vi "_Find Named Range.vi"(8 "error in":errorcluster, 9 "Sheet Name":string, 10 "Range Identifier":string, 11 "SpreadsheetDocument":refnum<k24>) -> (0 "error out":errorcluster, 1 "End Cell":cluster{"Col":string, "Row":i32}, 2 "Start Cell":cluster{"Col":string, "Row":i32}, 3 "SpreadsheetDocument":refnum<k24>, 4 "Sheet Name":string)   [LabVIEW 2021, in "Open Xml.lvlib"]
uses:
  Open Xml.lvlib
  D:/git/Open-Xml-LabVIEW/DocumentFormat.OpenXml.dll
  DocumentFormat.OpenXml.dll
  D:/git/Open-Xml-LabVIEW/DocumentFormat.OpenXml.Framework.dll
  DocumentFormat.OpenXml.Framework.dll
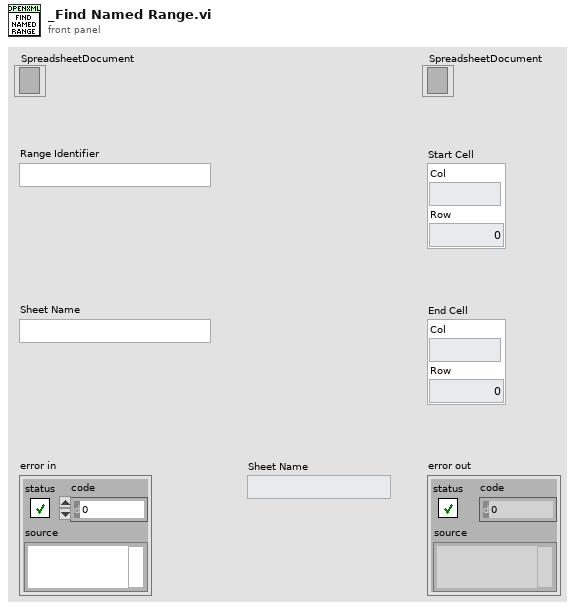
[diagram p1: front panel]
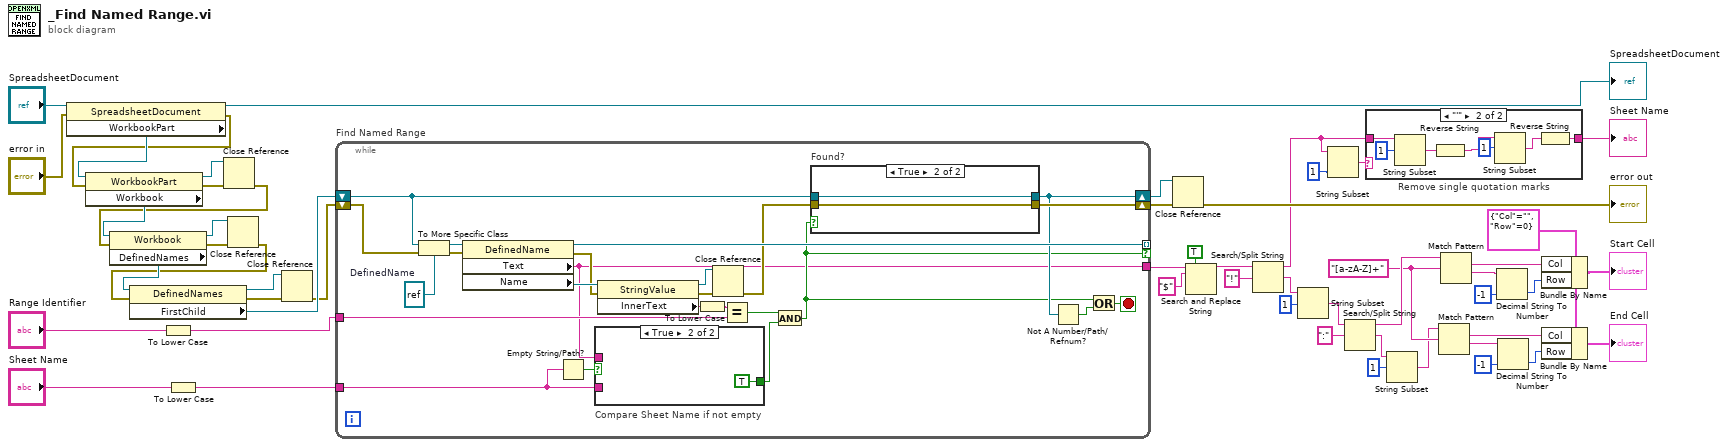
[diagram p0: block diagram]
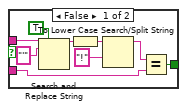
[diagram p2: hidden frame]
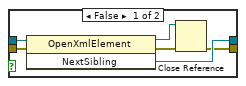
[diagram p3: hidden frame]
diagram:
  w26 = cluster{"Col":string, "Row":i32} {"Col"="", "Row"=0} ("input cluster")
  w28 = "[a-zA-Z]+" ("regular expression")
  n1 = property class="SpreadsheetDocument"(reference="SpreadsheetDocument", error in="error in") -> (reference out=→"SpreadsheetDocument":refnum<k24>, error out=w47:errorcluster, "WorkbookPart"=w52:refnum<k24>)
  n2 = property class="WorkbookPart"(reference=w52, error in=w47) -> (reference out=w14:refnum<k24>, error out=w46:errorcluster, "Workbook"=w53:refnum<k24>)
  n3 = To Lower Case(string="Range Identifier") -> (all lower case string=w1:string)
  n4 = To Lower Case(string="Sheet Name") -> (all lower case string=w2:string)
  n5 = Close Reference(reference=w14, error in (no error)=w46) -> (error out=w15:errorcluster)
  n6 = property class="Workbook"(reference=w53, error in=w15) -> (reference out=w12:refnum<k24>, error out=w45:errorcluster, "DefinedNames"=w51:refnum<k24>)
  n7 = Close Reference(reference=w12, error in (no error)=w45) -> (error out=w13:errorcluster)
  n8 = property class="DefinedNames"(reference=w51, error in=w13) -> (reference out=w10:refnum<k24>, error out=w50:errorcluster, "FirstChild"=w43:refnum<k24>)
  n9 = Close Reference(reference=w10, error in (no error)=w50) -> (error out=w11:errorcluster)
  n10 = while "Find Named Range" {
    shift-right: [w71] -> w44
    shift-left: w11 -> [w77]
    tunnel: [w73] -> _ mode=indexing if=w57
    tunnel: w1 -> [w68]
    tunnel: [w56] -> w40
    shift-right: [w62] -> w8
    shift-left: w43 -> [w63]
    tunnel: w2 -> [w58]
    stop <- w75 stop-if-true
    w65 = refnum<k24> refnum  # DefinedName
    n11 = To More Specific Class(target class=w65, reference=w63, error in=w77) -> (specific class reference=w74:refnum<k24>, error out=w72:errorcluster)
    n12 = property class="DefinedName"(reference=w74, error in=w72) -> (reference out=w73:refnum<k24>, error out=w69:errorcluster, "Text"=w56:string, "Name"=w70:refnum<k24>)
    n13 = Empty String/Path?(string/path=w58) -> (empty?=w59:bool)
    n14 = case "Compare Sheet Name if not empty" shown="True" w59 {
      tunnel: w58 -> [w81 _]
      tunnel: w56 -> [w82 _]
      tunnel: [w79 TRUE] -> w55
      frame False {
        n15 = Search and Replace String(replace all?=TRUE ("replace all? (F)"), input string=w82, search string="'") -> (result string=w86:string)  [unwired: 5 in, 3 out]
        n16 = To Lower Case(string=w86) -> (all lower case string=w80:string)
        n17 = Search/Split String(string=w80, search string/char (-)="!") -> (substring before match=w78:string)  [unwired: 1 in, 2 out]
        n18 = Equal?(x=w78, y=w81) -> (x = y?=w79:bool)
      }
      frame True {
      }
    }
    n19 = property class="StringValue"(reference=w70, error in=w69) -> (reference out=w60:refnum<k24>, error out=w67:errorcluster, "InnerText"=w64:string)
    n20 = To Lower Case(string=w64) -> (all lower case string=w54:string)
    n21 = Close Reference(reference=w60, error in (no error)=w67) -> (error out=w61:errorcluster)
    n22 = Equal?(x=w54, y=w68) -> (x = y?=w66:bool)
    n23 = And(x=w66, y=w55) -> (x .and. y?=w57:bool)
    n24 = case "Found?" shown="True" w57 {
      tunnel: [w89 w95] -> w71
      tunnel: w63 -> [w92 w94]
      tunnel: w61 -> [w91 w95]
      tunnel: [w90 w94] -> w62
      frame False {
        n25 = invoke class="OpenXmlElement" method="NextSibling"(reference=w92, error in=w91) -> (reference out=w88:refnum<k24>, error out=w93:errorcluster, "NextSibling"=w90:refnum<k24>)  [unwired: 1 in]
        n26 = Close Reference(reference=w88, error in (no error)=w93) -> (error out=w89:errorcluster)
      }
      frame True {
      }
    }
    n27 = Not A Number/Path/Refnum?(number/path/refnum=w62) -> (NaN/Path/Refnum?=w76:bool)
    n28 = Or(x=w57, y=w76) -> (x .or. y?=w75:bool)
  }
  n29 = Close Reference(reference=w8, error in (no error)=w44) -> (error out=→"error out":errorcluster)
  n30 = Search and Replace String(replace all?=TRUE ("replace all? (F)"), input string=w40, search string="$") -> (result string=w38:string)  [unwired: 5 in, 3 out]
  n31 = Search/Split String(string=w38, search string/char (-)="!") -> (substring before match=w5:string, match + rest of string=w36:string)  [unwired: 1 in, 1 out]
  n32 = String Subset(string=w36, offset (0)=1) -> (substring=w34:string)  [unwired: 1 in]
  n33 = String Subset(string=w5, length (rest)=1 ("length (rest)")) -> (substring=w4:string)  [unwired: 1 in]
  n34 = Search/Split String(string=w34, search string/char (-)=":") -> (substring before match=w31:string, match + rest of string=w32:string)  [unwired: 1 in, 1 out]
  n35 = case "Remove single quotation marks" shown="\"'\"" w4 {
    tunnel: [w96 w97] -> w7
    tunnel: w5 -> [w96 w103]
    frame Default {
    }
    frame "'" {
      n36 = String Subset(string=w103, offset (0)=1) -> (substring=w101:string)  [unwired: 1 in]
      n37 = Reverse String(1:w101) -> (0:w100:string)
      n38 = String Subset(string=w100, offset (0)=1) -> (substring=w99:string)  [unwired: 1 in]
      n39 = Reverse String(1:w99) -> (0:w97:string)
    }
  }
  "Sheet Name" <- w7
  n40 = String Subset(string=w32, offset (0)=1) -> (substring=w27:string)  [unwired: 1 in]
  n41 = Match Pattern(string=w27, regular expression=w28) -> (match substring=w16:string, after substring=w17:string)  [unwired: 1 in, 2 out]
  n42 = Match Pattern(string=w31, regular expression=w28) -> (match substring=w30:string, after substring=w29:string)  [unwired: 1 in, 2 out]
  n43 = Decimal String To Number(string=w29, default (0L)=-1 ("default (0 I32)")) -> (number=w18:i32)  [unwired: 1 in, 1 out]
  n44 = Decimal String To Number(string=w17, default (0L)=-1 ("default (0 I32)")) -> (number=w19:i32)  [unwired: 1 in, 1 out]
  n45 = Bundle By Name(cluster=w26, "Col"=w30, "Row"=w18) -> (→"Start Cell":cluster{"Col":string, "Row":i32})
  n46 = Bundle By Name(cluster=w26, "Col"=w16, "Row"=w19) -> (→"End Cell":cluster{"Col":string, "Row":i32})
